vi "Chart_Error_Prepare (SubVI).vi"(0 "Errors":string[](array[string]), 7 "Array in":dbl[](array[numeric]), 9 "Info":dbl, 11 "Value":dbl) -> (4 "RPM":dbl(graph), 6 "Velocity":dbl(graph), 8 "Coolant":dbl(graph), 10 "Engine Load":dbl(graph), 15 "Array out":string[](array[string]))   [LabVIEW 2017]
doc: "SubVI that decide basing on value of <B>Info</B> on which chart or table <B>Value</B> is to be displayed(Velocity, Clooland.RPM,Engine Load,Errors)."
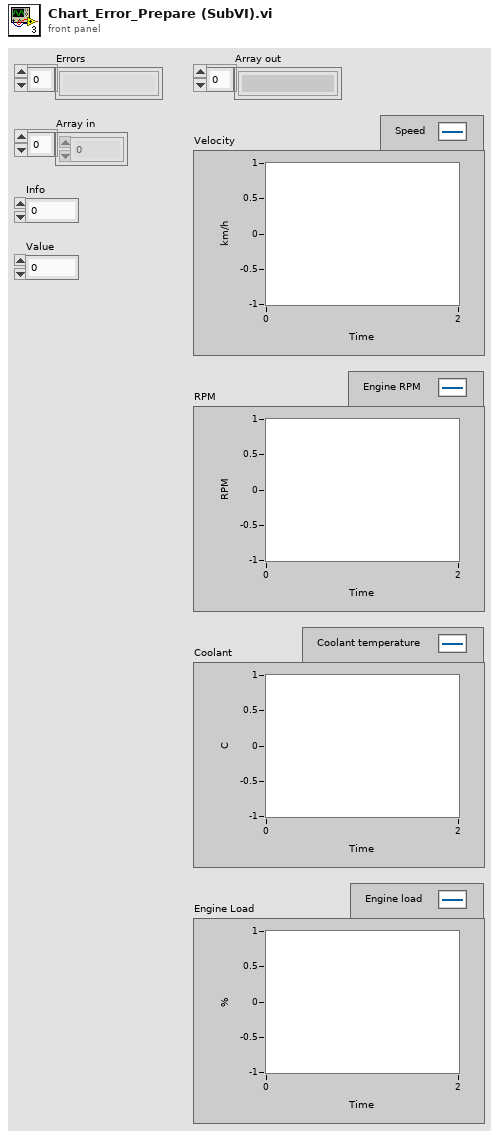
[diagram p1: front panel]
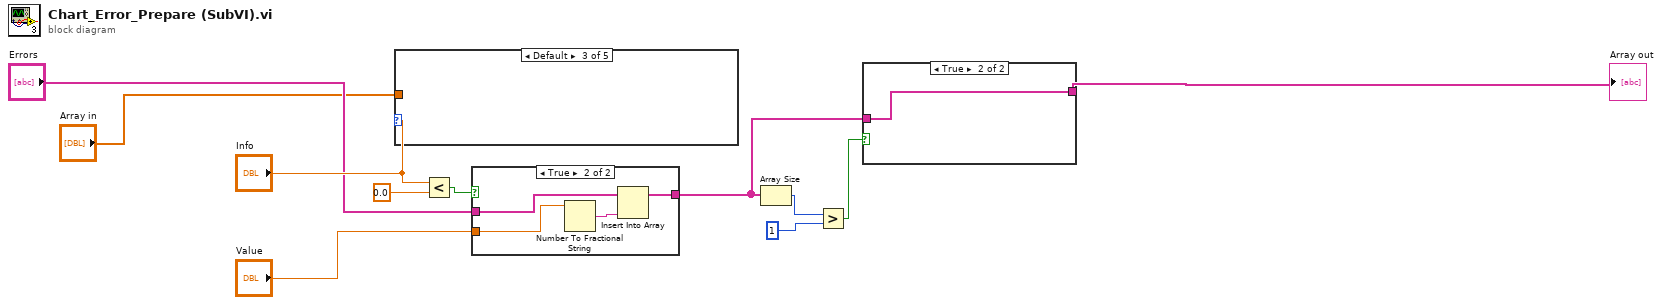
[diagram p0: block diagram]
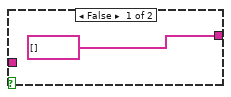
[diagram p2: hidden frame]
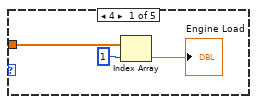
[diagram p4: hidden frame]
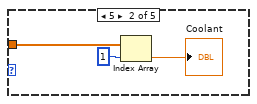
[diagram p5: hidden frame]
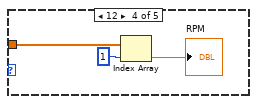
[diagram p6: hidden frame]
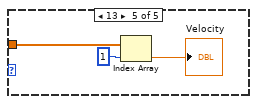
[diagram p7: hidden frame]
diagram:
  n1 = case shown="Default" "Info" {
    tunnel: "Array in" -> [w13 w16 _ w19 w22]
    frame 4 {
      n2 = Index Array(array=w13, index=1) -> (element=→"Engine Load":dbl)
    }
    frame 5 {
      n3 = Index Array(array=w16, index=1) -> (element=→"Coolant":dbl)
    }
    frame Default {
    }
    frame 12 {
      n4 = Index Array(array=w19, index=1) -> (element=→"RPM":dbl)
    }
    frame 13 {
      n5 = Index Array(array=w22, index=1) -> (element=→"Velocity":dbl)
    }
  }
  n6 = Less?(x="Info", y=0.0) -> (x < y?=w3:bool)
  n7 = case shown="True" w3 {
    tunnel: "Errors" -> [w24 w26]
    tunnel: "Value" -> [_ w28]
    tunnel: [w24 w25] -> w7
    frame False {
    }
    frame True {
      n8 = Number To Fractional String(number=w28) -> (F-format string=w27:string)  [unwired: 3 in]
      n9 = Insert Into Array(array=w26, new element=w27) -> (w25:string[])  [unwired: 1 in]
    }
  }
  n10 = Array Size(array=w7) -> (size(s)=w8:i32)
  n11 = Greater?(x=w8, y=1) -> (0:w10:bool)
  n12 = case shown="True" w10 {
    tunnel: w7 -> [_ w30]
    tunnel: [string[] [] w30] -> w11
    frame False {
    }
    frame True {
    }
  }
  "Array out" <- w11
